vi "updateFieldnumber - subvi.vi"(9 "Field Size":dbl, 10 "CurY":dbl, 11 "CurX":dbl) -> (3 "Field Number":u32)   [LabVIEW 2014]
uses:
  stage-controller-globals.vi
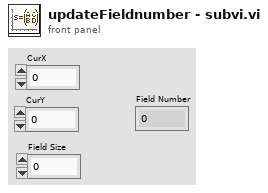
[diagram p1: front panel]
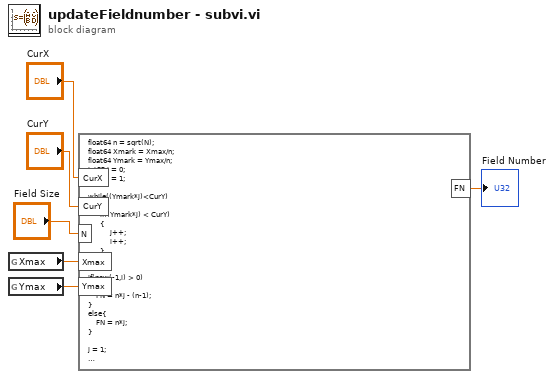
[diagram p0: block diagram]
diagram:
  n1 = global read "stage-controller-globals.vi" "Xmax"() -> (w5:dbl)
  n2 = global read "stage-controller-globals.vi" "Ymax"() -> (w6:dbl)
  n3 = formula code="float64 n = sqrt(N);\nfloat64 Xmark = Xmax/n;\nfloat64 Ymark = Ymax/n;\nint32 i = 0;\nint32 j = 1;\n\nwhile((Ymark*j)<CurY)\n{\n      if((Ymark*j) < CurY)\n      {\n           j++;\n           i++;\n      }\n}\n\nif(pow(-1,i) > 0)\n{\n    FN = n*j - (n-1);\n}\nelse{\n    FN = n*j;\n}\n\nj = 1;\n\nwhile((Xmark*j) < CurX)\n{\n    if((Xmark*j) <CurX)\n    {\n         FN = FN + pow(-1,i);\n         j++;\n    }\n}"("CurX"="CurX", "CurY"="CurY", "N"="Field Size", "Xmax"=w5, "Ymax"=w6) -> ("FN"=→"Field Number":dbl)
